vi "Advanced Copy (No Check).vi"(0 "src Pointer in":refnum<class "Pointer.lvclass">, 1 "dst width":u64 format="%d bytes", 2 "src width":u64 format="%d bytes", 5 "dst Pointer in":refnum<class "Pointer.lvclass">, 7 "src offset (0)":u64 format="%d bytes", 9 "dst offset (0)":u64 format="%d bytes", 11 "error in (no error)":errorcluster, 12 "src byte order (little-endian)":enum16{"big-endian", "little-endian"}(ring)=enum."little-endian", 13 "dst byte order (little-endian)":enum16{"big-endian", "little-endian"}(ring)=enum."little-endian", 14 "clear dst bytes? (T)":bool=TRUE) -> (4 "src Pointer out":refnum<class "Pointer.lvclass">, 6 "dst Pointer out":refnum<class "Pointer.lvclass">, 15 "error out":errorcluster)   [LabVIEW 2016, in "Memory Manager.lvlib" / "Pointer.lvclass"]
doc: "Moves bytes of data from the <b>src pointer</b> at <b>src offset</b> to the <b>dst pointer</b> at <b>dst offset</b> using the <b>byte order</b> specified. <b>src width</b> and <b>dst width</b> are used to determine how many bytes to move, as well as where the bytes should be read from/written to in memory. For example, to type cast a DBL to a U16, src width would be 8 bytes and dst width would be 2 bytes.\n\nThe optional argument <b>clear dst bytes</b> will clear the subset of bytes within <b>dst pointer</b> before moving data from the <b>src pointer</b>. This is required when type casting from a smaller type to a larger type, as the larger type may have non-zero bytes that will not get overwritten. This argument can be set the FALSE when casting larger types down to smaller types.\n\n<b>Note:</b> This VI is <b>unsafe</b>, meaning it does not performs null pointer and bounds checks to prevent invalid memory access. Invalid arguments provided to this method can crash or corrupt LabVIEW memory."
uses:
  Pointer.lvclass
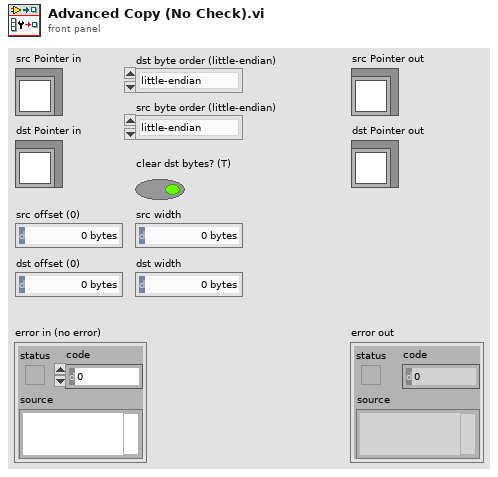
[diagram p1: front panel]
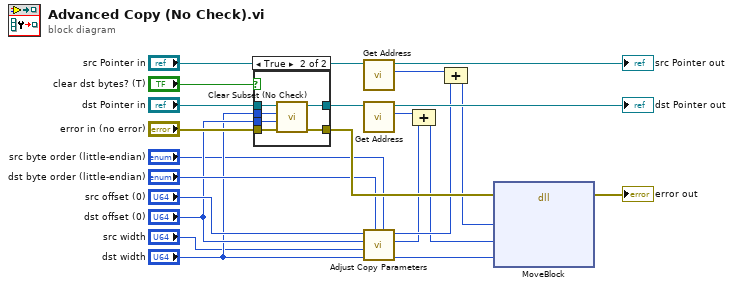
[diagram p0: block diagram]
diagram:
  n1 = case shown="True" "clear dst bytes? (T)" {
    tunnel: [w23 w30] -> w22
    tunnel: "error in (no error)" -> [w23 w29]
    tunnel: "dst Pointer in" -> [w24 w28]
    tunnel: [w24 w27] -> w9
    tunnel: "dst offset (0)" -> [_ w26]
    tunnel: "dst width" -> [_ w25]
    frame False {
    }
    frame True {
      n2 = call "Clear Subset (No Check).vi"("error in (no error)"=w29, "offset (0)"=w26, "length (-1: rest)"=w25, "Pointer in"=w28) -> ("error out"=w30:errorcluster, "Pointer out"=w27:refnum<class "Pointer.lvclass">)  [unwired: 6 in]
    }
  }
  n3 = call "Get Address.vi"("Pointer in"="src Pointer in") -> ("address"=w13:u64, "Pointer out"=→"src Pointer out":refnum<class "Pointer.lvclass">)  [unwired: 9 in]
  n4 = call "Get Address.vi"("Pointer in"=w9) -> ("address"=w8:u64, "Pointer out"=→"dst Pointer out":refnum<class "Pointer.lvclass">)  [unwired: 9 in]
  n5 = call "Adjust Copy Parameters.vi"("src byte order (little-endian)"="src byte order (little-endian)", "dst byte order (little-endian)"="dst byte order (little-endian)", "dst width"="dst width", "src width"="src width", "dst offset in"="dst offset (0)", "src offset in"="src offset (0)") -> ("bytes to move"=w15:u64, "dst offset out"=w7:u64, "src offset out"=w12:u64)  [unwired: 2 in, 1 out]
  n6 = Compound Arithmetic op=ADD(w8, w7) -> (w6:u64)
  n7 = Compound Arithmetic op=ADD(w13, w12) -> (w11:u64)
  n8 = dll-call lib="LabVIEW" fn="MoveBlock"(error in=w22, "src"=w11, "dst"=w6, "size"=w15) -> (error out=→"error out":errorcluster)  [unwired: 6 in, 1 out]
